vi "Create.vi"(8 "error in (no error)":errorcluster, 10 "DLL path":path) -> (0 "error out":errorcluster, 3 "Skeleton out":refnum<class "Skeleton.lvclass">)   [LabVIEW 2016, in "Skeleton.lvlib" / "Skeleton.lvclass"]
uses:
  Skeleton.lvclass
  Private Data.ctl
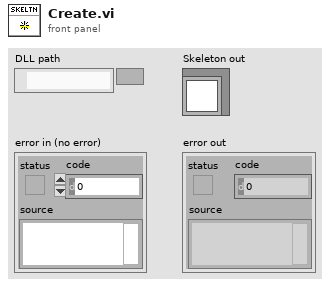
[diagram p1: front panel]
types:
  T1 = typedef "Skeleton.lvlib/Skeleton.lvclass/Private Data.ctl" = cluster{"DLL path":path}
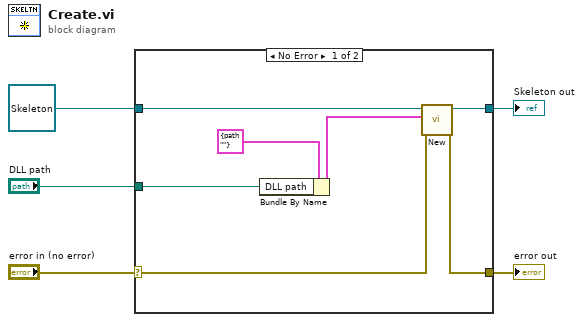
[diagram p0: block diagram]
diagram:
  n1 = case shown="No Error" "error in (no error)" {
    selector: "error in (no error)" -> [w10 w14]
    tunnel: [w9 w14] -> w4
    tunnel: refnum<class "Skeleton.lvclass"> refnum ("Skeleton out") -> [w12 w13]
    tunnel: [w11 w13] -> w2
    tunnel: "DLL path" -> [w6 _]
    frame No Error {
      n2 = Bundle By Name(cluster=T1 {"DLL path"=path ""} ("Private Data"), "DLL path"=w6) -> (w7:T1)
      n3 = call "New.vi"("error in (no error)"=w10, "Private Data"=w7, "Skeleton in"=w12) -> ("error out"=w9:errorcluster, "Skeleton out"=w11:refnum<class "Skeleton.lvclass">)  [unwired: 7 in]
    }
    frame Error {
    }
  }
  "error out" <- w4
  "Skeleton out" <- w2
